vi "Remote Control.vi"(7 "Calling VI Ref":refnum<vi>) -> ()   [LabVIEW 2020]
uses:
  <vilib>/Utility/miscctls.llb/LVPointTypeDef.ctl
  Remote Control Type Defs/Remote Control Actions.ctl
  4Pi Dual DM Control/4Pi Dual DM - Controls/4Pi Dual DM - Standard Action.ctl
panel:
  out "Error":bool
  out "Connected":bool
  in  "Quit":bool
  out "Port":u16=1
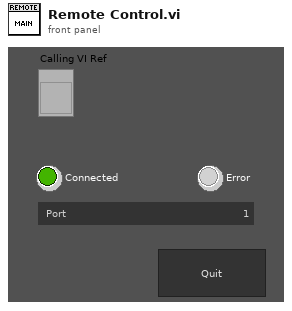
[diagram p1: front panel]
types:
  T1 = typedef "Remote Control Actions.ctl" = enum16{"Listen", "Wait Cmd", "Set Ctrl Values", "Get Ctrl Values", "Start Live", "Get Image", "Stop Live", "Quit"}
  T2 = enum16{"Always On", "Always Off", "Off While Running"}
  T3 = typedef "LVPointTypeDef.ctl" = cluster{"Horizontal":i16, "Vertical":i16}
  T4 = typedef "4Pi Dual DM - Standard Action.ctl" = enum16{"Read", "Write"}
  T5 = typedef "4Pi Dual DM - Mirror Modes DUAL.ctl" = cluster{"Mode":string, "Amplitude":dbl}[][]
  T6 = typedef "LVRectTypeDef.ctl" = cluster{"Left":i16, "Top":i16, "Right":i16, "Bottom":i16}
  T7 = typedef "LVBoundsTypeDef.ctl" = cluster{"Width":u32, "Height":u32}
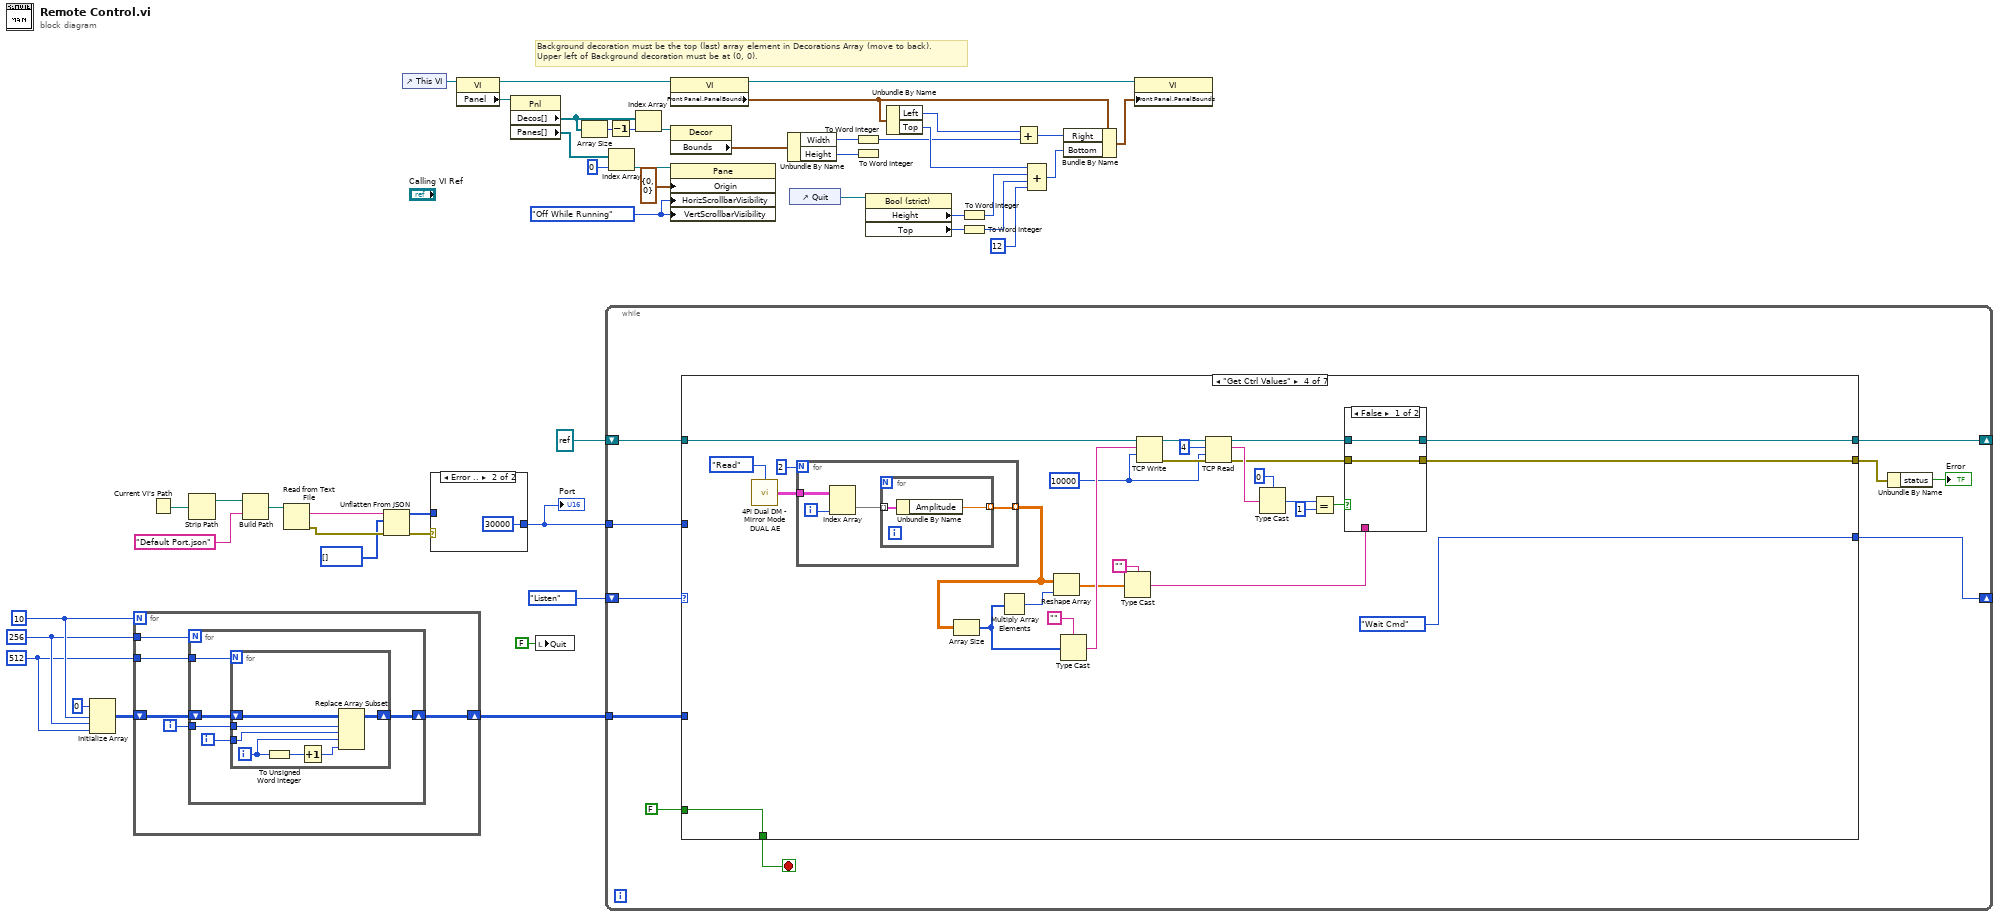
[diagram p0: block diagram]
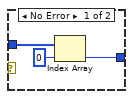
[diagram p2: hidden frame]
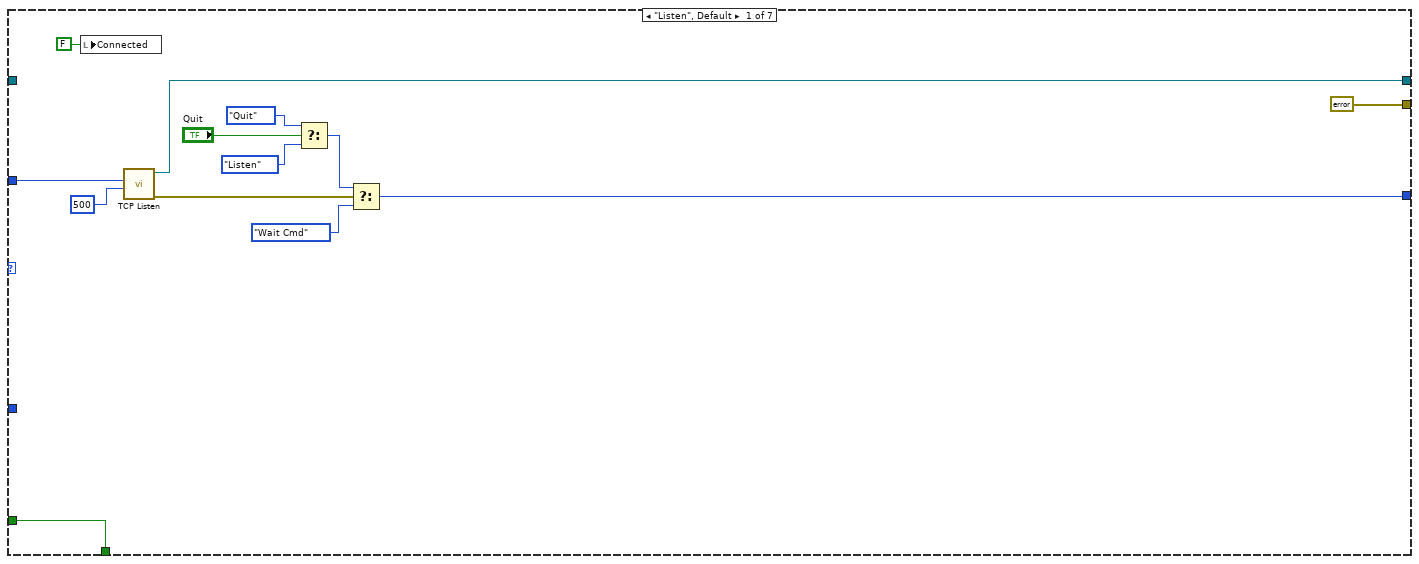
[diagram p3: hidden frame]
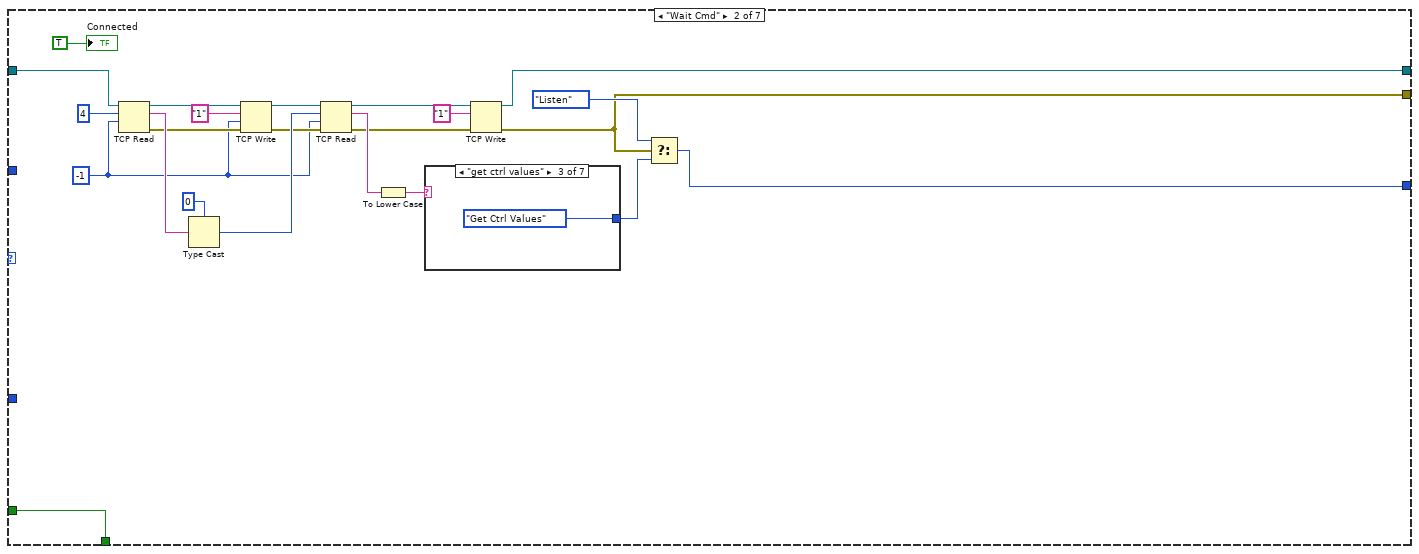
[diagram p4: hidden frame]
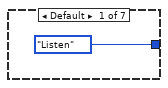
[diagram p5: hidden frame]
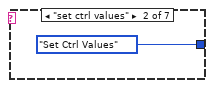
[diagram p6: hidden frame]
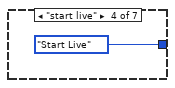
[diagram p7: hidden frame]
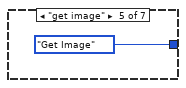
[diagram p8: hidden frame]
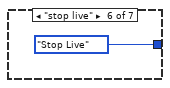
[diagram p9: hidden frame]
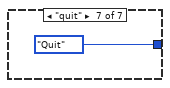
[diagram p10: hidden frame]
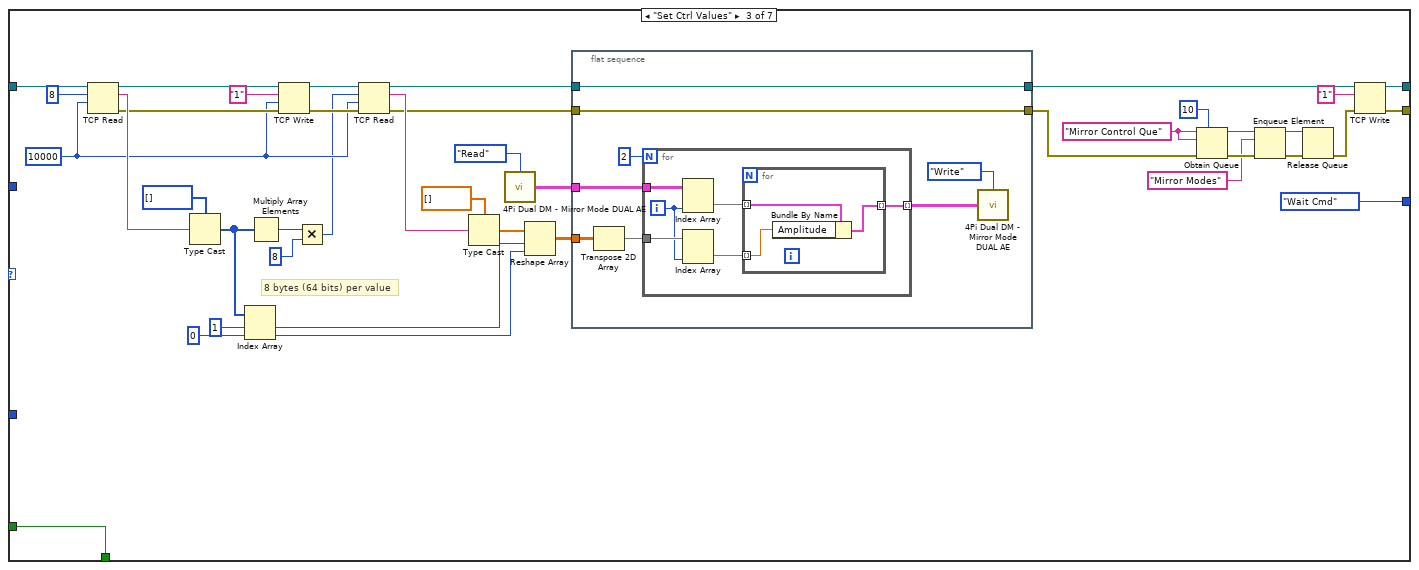
[diagram p11: hidden frame]
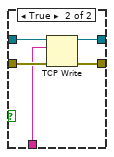
[diagram p12: hidden frame]
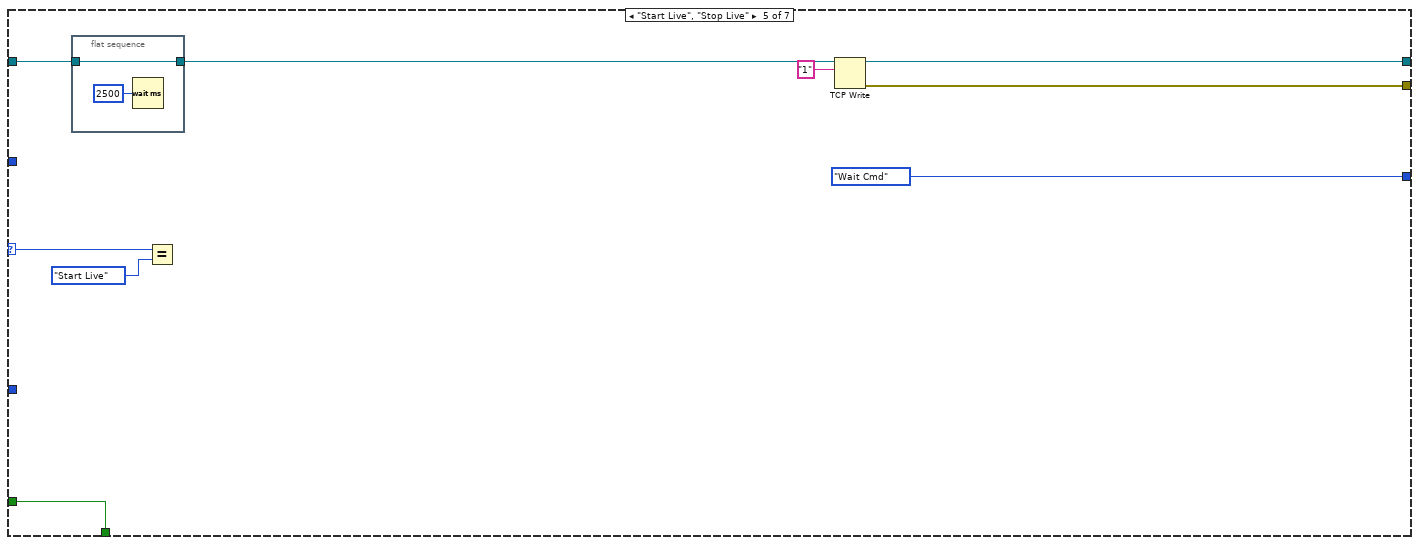
[diagram p13: hidden frame]
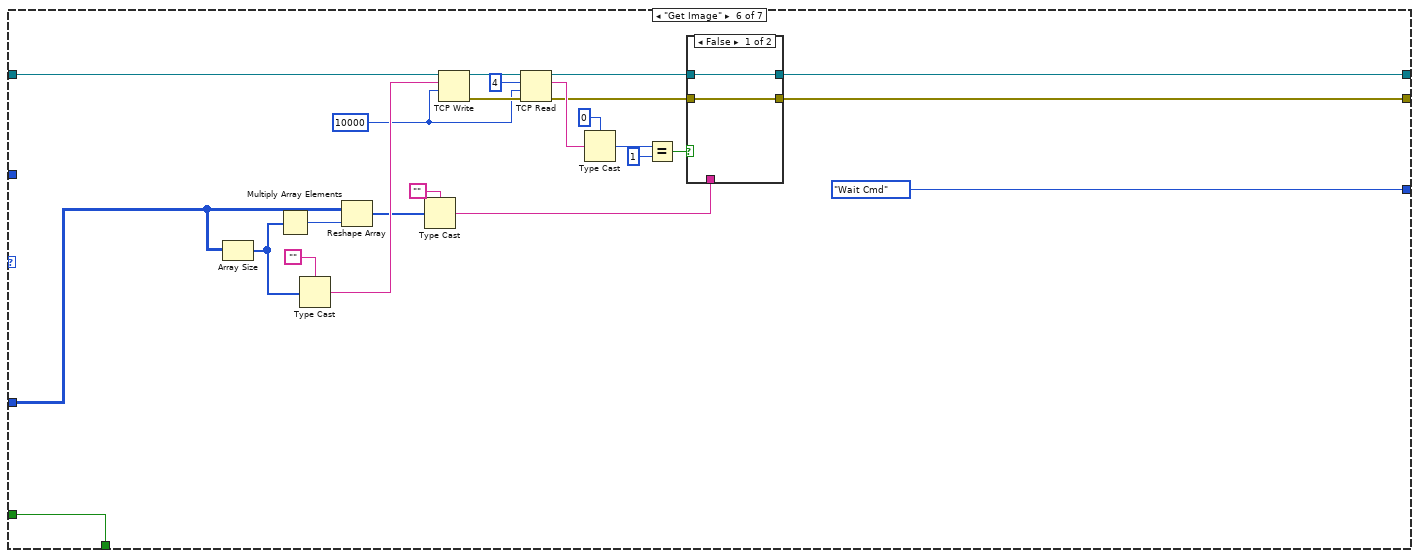
[diagram p14: hidden frame]
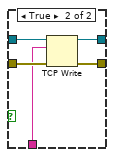
[diagram p15: hidden frame]
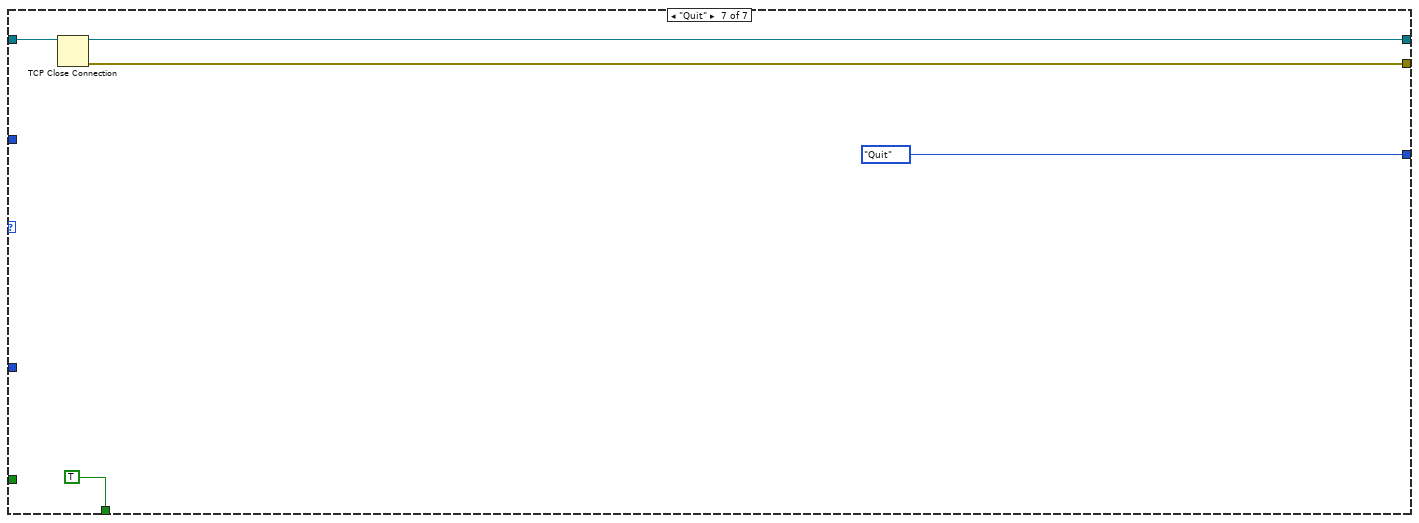
[diagram p16: hidden frame]
diagram:
  w4 = 512
  w5 = 256
  w6 = 10
  w31 = T2."Off While Running" ("Vertical Scrollbar Visibility")
  # "Background decoration must be the top (last) array element in Decorations Array (move to back).\nUpper left of Background decoration must be at (0, 0)."
  n1 = Initialize Array(u16 0 ("element"), w6, w5, w4) -> (w3:u16[][][])
  n2 = for {
    N: w6 -> [_]
    tunnel: w5 -> [w53]
    tunnel: w4 -> [w52]
    shift-right: [w49] -> w1
    shift-left: w3 -> [w51]
    i -> [w50]
    n3 = for {
      N: w53 -> [_]
      tunnel: w52 -> [w58]
      shift-right: [w54] -> w49
      shift-left: w51 -> [w57]
      tunnel: w50 -> [w56]
      i -> [w55]
      n4 = for {
        N: w58 -> [_]
        shift-right: [w59] -> w54
        shift-left: w57 -> [w65]
        tunnel: w56 -> [w64]
        tunnel: w55 -> [w63]
        i -> [w61]
        n5 = To Unsigned Word Integer(number=w61) -> (unsigned 16bit integer=w60:u16)
        n6 = Increment(x=w60) -> (x+1=w62:u16)
        n7 = Replace Array Subset(array=w65, new element=w62, index (dim 0)=w64, index (dim 1)=w63, index (dim 2)=w61) -> (w59:u16[][][])
      }
    }
  }
  n8 = Current VI's Path() -> (path=w19:path)
  n9 = Strip Path(path=w19) -> (stripped path=w18:path)  [unwired: 1 out]
  n10 = Build Path(base path=w18, name or relative path="Default Port.json") -> (appended path=w16:path)
  n11 = Read from Text File(file (use dialog)=w16) -> (text=w15:string, error out=w14:errorcluster)  [unwired: 3 in, 2 out]
  n12 = Unflatten From JSON(JSON string=w15, type and defaults=u16[] [], error in (no error)=w14) -> (value=w12:u16[], error out=w13:errorcluster)  [unwired: 4 in]
  n13 = control-ref of="This VI"() -> (w23:refnum<vi>)
  n14 = case shown="Error .." w13 {
    tunnel: w12 -> [w68 _]
    tunnel: [w66 u16 30000] -> w8
    frame No Error {
      n15 = Index Array(array=w68, index=0) -> (element=w66:u16)
    }
    frame Error {
    }
  }
  "Port" <- w8
  n16 = property class="VI"(reference=w23) -> (reference out=w32:refnum<vi>, "Panel"=w24:refnum<vi>)  [unwired: 1 in, 1 out]
  n17 = property class="Pnl"(reference=w24) -> ("Decos[]"=w22:refnum<vi>[], "Panes[]"=w28:refnum<vi>[])  [unwired: 1 in, 2 out]
  n18 = local write "Quit"(FALSE ("Quit")) -> ()
  n19 = Array Size(array=w22) -> (size(s)=w20:i32)
  n20 = while {
    shift-right: [w75] -> _
    shift-left: refnum<k5> refnum ("connection ID") -> [w79]
    shift-right: [w77] -> _
    shift-left: Remote_Control_Actions."Listen" ("Remote Action") -> [w78]
    tunnel: w8 -> [w76]
    tunnel: w1 -> [w72]
    stop <- w74 stop-if-true
    n21 = case shown="\"Get Ctrl Values\"" w78 {
      selector: w78 -> [_ _ _ _ w228 _ _]
      tunnel: w79 -> [_ w100 w153 w204 w223 w236 w265]
      tunnel: w76 -> [w92 _ _ _ _ _ _]
      tunnel: [w83 w97 Remote_Control_Actions."Wait Cmd" ("Remote Action") Remote_Control_Actions."Wait Cmd" ("Remote Action") Remote_Control_Actions."Wait Cmd" ("Remote Action") Remote_Control_Actions."Wait Cmd" ("Remote Action") Remote_Control_Actions."Quit" ("Remote Action")] -> w77
      tunnel: [w86 w99 w152 w191 w225 w234 w264] -> w75
      tunnel: [w91 w115 w163 w207 w229 w255 TRUE] -> w74
      tunnel: FALSE -> [w91 w115 w163 w207 w229 w255 _]
      tunnel: w72 -> [_ _ _ _ _ w233 _]
      tunnel: [errorcluster {"status"=FALSE, "code"=0, "source"=""} ("error out") w93 w138 w184 w221 w232 w263] -> w71
      frame "Listen", Default {
        n22 = local write "Connected"(FALSE ("Connected")) -> ()
        n23 = call <vilib>:"TCP Listen.vi"("timeout ms (wait forever: -1)"=500, "port"=w92) -> ("error out"=w81:errorcluster, "connection ID"=w86:refnum<k5>)  [unwired: 5 in, 3 out]
        n24 = Select(t=Remote_Control_Actions."Quit" ("Remote Action"), s="Quit", f=Remote_Control_Actions."Listen" ("Remote Action")) -> (s? t:f=w85:T1)
        n25 = Select(t=w85, s=w81, f=Remote_Control_Actions."Wait Cmd" ("Remote Action")) -> (s? t:f=w83:T1)
      }
      frame "Wait Cmd" {
        w103 = -1 ("timeout ms (wait forever: -1)")
        n26 = TCP Read(connection ID=w100, bytes to read=4, 9:w103) -> (connection ID out=w106:refnum<k5>, data out=w110:string, error out=w107:errorcluster)  [unwired: 2 in]
        n27 = Type Cast(type=0 ("bytes to read"), x=w110) -> (*(type *) &x=w111:i32)
        n28 = TCP Write(connection ID=w106, data in="1", error in (no error)=w107, 9:w103) -> (connection ID out=w108:refnum<k5>, error out=w109:errorcluster)  [unwired: 1 out]
        n29 = TCP Read(connection ID=w108, bytes to read=w111, error in (no error)=w109, 9:w103) -> (connection ID out=w112:refnum<k5>, data out=w114:string, error out=w113:errorcluster)  [unwired: 1 in]
        n30 = To Lower Case(string=w114) -> (all lower case string=w95:string)
        n31 = case shown="\"get ctrl values\"" w95 {
          tunnel: [Remote_Control_Actions."Listen" ("Remote Action") Remote_Control_Actions."Set Ctrl Values" ("Remote Action") Remote_Control_Actions."Get Ctrl Values" ("Remote Action") Remote_Control_Actions."Start Live" ("Remote Action") Remote_Control_Actions."Get Image" ("Remote Action") Remote_Control_Actions."Stop Live" ("Remote Action") Remote_Control_Actions."Quit" ("Remote Action")] -> w98
          frame Default {
          }
          frame "set ctrl values" {
          }
          frame "get ctrl values" {
          }
          frame "start live" {
          }
          frame "get image" {
          }
          frame "stop live" {
          }
          frame "quit" {
          }
        }
        n32 = TCP Write(connection ID=w112, data in="1", error in (no error)=w113) -> (connection ID out=w99:refnum<k5>, error out=w93:errorcluster)  [unwired: 1 in, 1 out]
        n33 = Select(t=Remote_Control_Actions."Listen" ("Remote Action"), s=w93, f=w98) -> (s? t:f=w97:T1)
        "Connected" <- TRUE ("Connected")
      }
      frame "Set Ctrl Values" {
        w127 = "Mirror Control Que" ("name (unnamed)")
        w156 = 10000 ("timeout ms (wait forever: -1)")
        # "8 bytes (64 bits) per value"
        n34 = TCP Read(connection ID=w153, bytes to read=8, 9:w156) -> (connection ID out=w158:refnum<k5>, data out=w162:string, error out=w159:errorcluster)  [unwired: 2 in]
        n35 = Type Cast(type=i32[] [], x=w162) -> (*(type *) &x=w144:i32[])
        n36 = Index Array(array=w144, index #1=1 ("index"), index #2=0 ("index")) -> (element #1=w141:i32, element #2=w140:i32)
        n37 = Multiply Array Elements(1:w144) -> (0:w148:i32)
        n38 = TCP Write(connection ID=w158, data in="1", error in (no error)=w159, 9:w156) -> (connection ID out=w160:refnum<k5>, error out=w161:errorcluster)  [unwired: 1 out]
        n39 = Multiply(x=w148, y=8) -> (x*y=w150:i32)
        n40 = TCP Read(connection ID=w160, bytes to read=w150, error in (no error)=w161, 9:w156) -> (connection ID out=w134:refnum<k5>, data out=w146:string, error out=w133:errorcluster)  [unwired: 1 in]
        n41 = Type Cast(type=dbl[] [], x=w146) -> (*(type *) &x=w145:dbl[])
        n42 = call "4Pi Dual DM - Mirror Mode DUAL AE.vi"("Action"=4Pi_Dual_DM_-_Standard_Action."Read") -> ("Mirror Modes Out"=w137:T5)  [unwired: 14 in]
        n43 = Reshape Array(w145, w141, w140) -> (w139:dbl[][])
        n44 = flat-sequence {
          tunnel: w139 -> [w171]
          tunnel: w137 -> [w169]
          tunnel: w134 -> [w165]
          tunnel: [w165] -> w125
          tunnel: w133 -> [w164]
          tunnel: [w164] -> w124
          frame #0 {
            n45 = Transpose 2D Array(2D array=w171) -> (transposed array=w166:dbl[][])
            n46 = for {
              N: 2 -> [_]
              tunnel: w169 -> [w177]
              tunnel: w166 -> [w175]
              tunnel: [w172] -> w170 mode=indexing
              i -> [w174]
              n47 = Index Array(array=w177, index (col)=w174) -> (element=w176:cluster{"Mode":string, "Amplitude":dbl}[])  [unwired: 1 in]
              n48 = Index Array(array=w175, index (col)=w174) -> (element=w173:dbl[])  [unwired: 1 in]
              n49 = for {
                tunnel: w176 -> [w180] mode=indexing
                tunnel: w173 -> [w179] mode=indexing
                tunnel: [w178] -> w172 mode=indexing
                n50 = Bundle By Name(cluster=w180, "Amplitude"=w179) -> (w178:cluster{"Mode":string, "Amplitude":dbl})
              }
            }
            n51 = call "4Pi Dual DM - Mirror Mode DUAL AE.vi"("Action"=4Pi_Dual_DM_-_Standard_Action."Write", "Mirror Modes In"=w170) -> ()  [unwired: 13 in, 1 out]
          }
        }
        n52 = Obtain Queue(max queue size (-1, unlimited)=10, name (unnamed)=w127, element data type=w127, error in (no error)=w124) -> (queue out=w130:refnum<queue>, error out=w131:errorcluster)  [unwired: 1 in, 1 out]
        n53 = Enqueue Element(queue=w130, element="Mirror Modes", error in (no error)=w131) -> (queue out=w129:refnum<queue>, error out=w132:errorcluster)  [unwired: 1 in, 1 out]
        n54 = Release Queue(queue=w129, error in (no error)=w132) -> (error out=w123:errorcluster)  [unwired: 1 in, 2 out]
        n55 = TCP Write(connection ID=w125, data in="1", error in (no error)=w123) -> (connection ID out=w152:refnum<k5>, error out=w138:errorcluster)  [unwired: 1 in, 1 out]
      }
      frame "Get Ctrl Values" {
        w199 = 10000 ("timeout ms (25000)")
        n56 = call "4Pi Dual DM - Mirror Mode DUAL AE.vi"("Action"=4Pi_Dual_DM_-_Standard_Action."Read") -> ("Mirror Modes Out"=w182:T5)  [unwired: 14 in]
        n57 = for {
          N: 2 -> [_]
          tunnel: w182 -> [w211]
          tunnel: [w208] -> w186 mode=indexing
          i -> [w210]
          n58 = Index Array(array=w211, index (col)=w210) -> (element=w209:cluster{"Mode":string, "Amplitude":dbl}[])  [unwired: 1 in]
          n59 = for {
            tunnel: w209 -> [w213] mode=indexing
            tunnel: [w212] -> w208 mode=indexing
            n60 = Unbundle By Name(w213) -> ("Amplitude"=w212:dbl)
          }
        }
        n61 = Array Size(array=w186) -> (size(s)=w185:i32[])
        n62 = Multiply Array Elements(1:w185) -> (0:w205:i32)
        n63 = Reshape Array(w186, w205) -> (w187:dbl[])
        n64 = Type Cast(type="", x=w185) -> (*(type *) &x=w201:string)
        n65 = Type Cast(type="", x=w187) -> (*(type *) &x=w188:string)
        n66 = TCP Write(connection ID=w204, data in=w201, 9:w199) -> (connection ID out=w202:refnum<k5>, error out=w200:errorcluster)  [unwired: 1 in, 1 out]
        n67 = TCP Read(connection ID=w202, bytes to read=4, error in (no error)=w200, 9:w199) -> (connection ID out=w192:refnum<k5>, data out=w196:string, error out=w190:errorcluster)  [unwired: 1 in]
        n68 = Type Cast(type=0 ("bytes to read"), x=w196) -> (*(type *) &x=w195:i32)
        n69 = Equal?(x=w195, y=1) -> (x = y?=w193:bool)
        n70 = case shown="False" w193 {
          tunnel: w192 -> [w215 w220]
          tunnel: [w215 w219] -> w191
          tunnel: w190 -> [w214 w218]
          tunnel: w188 -> [_ w217]
          tunnel: [w214 w216] -> w184
          frame False {
          }
          frame True {
            n71 = TCP Write(connection ID=w220, data in=w217, error in (no error)=w218) -> (connection ID out=w219:refnum<k5>, error out=w216:errorcluster)  [unwired: 1 in, 1 out]
          }
        }
      }
      frame "Start Live", "Stop Live" {
        n72 = flat-sequence {
          tunnel: w223 -> [w231]
          tunnel: [w231] -> w222
          frame #0 {
            n73 = Wait (ms)(milliseconds to wait=u32 2500) -> ()  [unwired: 1 out]
          }
        }
        n74 = Equal?(x=w228, y=Remote_Control_Actions."Start Live") -> ()  [unwired: 1 out]
        n75 = TCP Write(connection ID=w222, data in="1") -> (connection ID out=w225:refnum<k5>, error out=w221:errorcluster)  [unwired: 2 in, 1 out]
      }
      frame "Get Image" {
        w248 = 10000 ("timeout ms (25000)")
        n76 = Array Size(array=w233) -> (size(s)=w251:i32[])
        n77 = Multiply Array Elements(1:w251) -> (0:w254:i32)
        n78 = Type Cast(type="", x=w251) -> (*(type *) &x=w250:string)
        n79 = Reshape Array(w233, w254) -> (w237:u16[])
        n80 = Type Cast(type="", x=w237) -> (*(type *) &x=w238:string)
        n81 = TCP Write(connection ID=w236, data in=w250, 9:w248) -> (connection ID out=w252:refnum<k5>, error out=w249:errorcluster)  [unwired: 1 in, 1 out]
        n82 = TCP Read(connection ID=w252, bytes to read=4, error in (no error)=w249, 9:w248) -> (connection ID out=w241:refnum<k5>, data out=w245:string, error out=w240:errorcluster)  [unwired: 1 in]
        n83 = Type Cast(type=0 ("bytes to read"), x=w245) -> (*(type *) &x=w244:i32)
        n84 = Equal?(x=w244, y=1) -> (x = y?=w242:bool)
        n85 = case shown="False" w242 {
          tunnel: w241 -> [w257 w262]
          tunnel: [w257 w261] -> w234
          tunnel: w240 -> [w256 w260]
          tunnel: w238 -> [_ w259]
          tunnel: [w256 w258] -> w232
          frame False {
          }
          frame True {
            n86 = TCP Write(connection ID=w262, data in=w259, error in (no error)=w260) -> (connection ID out=w261:refnum<k5>, error out=w258:errorcluster)  [unwired: 1 in, 1 out]
          }
        }
      }
      frame "Quit" {
        n87 = TCP Close Connection(connection ID=w265) -> (connection ID out=w264:refnum<k5>, error out=w263:errorcluster)  [unwired: 2 in]
      }
    }
    n88 = Unbundle By Name(w71) -> ("status"=→"Error":bool)
  }
  n89 = Decrement(x=w20) -> (x-1=w21:i32)
  n90 = Index Array(array=w28, index=0) -> (element=w27:refnum<vi>)
  n91 = Index Array(array=w22, index=w21) -> (element=w30:refnum<vi>)
  n92 = property class="VI"(reference=w32) -> (reference out=w34:refnum<vi>, "Front Panel.PanelBounds"=w35:T6)  [unwired: 1 in, 1 out]
  n93 = property class="Decor"(reference=w30) -> ("Bounds"=w33:T7)  [unwired: 1 in, 2 out]
  n94 = property class="Pane"(reference=w27, "Origin"=T3 {"Horizontal"=0, "Vertical"=0}, "HorizScrollbarVisibility"=w31, "VertScrollbarVisibility"=w31) -> ()  [unwired: 1 in, 2 out]
  n95 = Unbundle By Name(w33) -> ("Width"=w38:u32, "Height"=w41:u32)
  n96 = control-ref of="Quit"() -> (w25:refnum<vi>)
  n97 = To Word Integer(number=w38) -> (16bit integer=w40:i16)
  n98 = To Word Integer(number=w41) -> ()  [unwired: 1 out]
  n99 = property class="Bool (strict)"(reference=w25) -> ("Height"=w43:u32, "Top"=w44:i32)  [unwired: 1 in, 2 out]
  n100 = Unbundle By Name(w35) -> ("Left"=w37:i16, "Top"=w48:i16)
  n101 = To Word Integer(number=w43) -> (16bit integer=w46:i16)
  n102 = To Word Integer(number=w44) -> (16bit integer=w47:i16)
  n103 = Add(x=w37, y=w40) -> (x+y=w39:i16)
  n104 = Compound Arithmetic op=ADD(w48, w46, w47, i16 12 ("y")) -> (w42:i16)
  n105 = Bundle By Name(cluster=w35, "Right"=w39, "Bottom"=w42) -> (w36:T6)
  n106 = property class="VI"(reference=w34, "Front Panel.PanelBounds"=w36) -> ()  [unwired: 1 in, 2 out]
